vi "acq.Video.vi"(7 "DVR":T3, 8 "error in":errorcluster, 9 "video":T2=TRUE caption="Save Video", 10 "buffer in":u16[][](array[numeric])) -> (0 "error out":errorcluster, 2 "AVI Refnum":T1)   [LabVIEW 2020]
uses:
  _controls/data.ctl
  camera/camera.lvclass
  _controls/data.ref.ctl
  <vilib>/vision/Image Controls.llb/IMAQ Image.ctl
  _controls/state.ctl
  _controls/data.vars.ctl
  _controls/flip.ctl
  _controls/checkbox.ctl
  <vilib>/vision/Avi.llb/IMAQ AVI2 Refnum.ctl
  pix.sgl.CalcPercentiles.sgl.vi
  pix.sgl.CalcPercentiles.vi
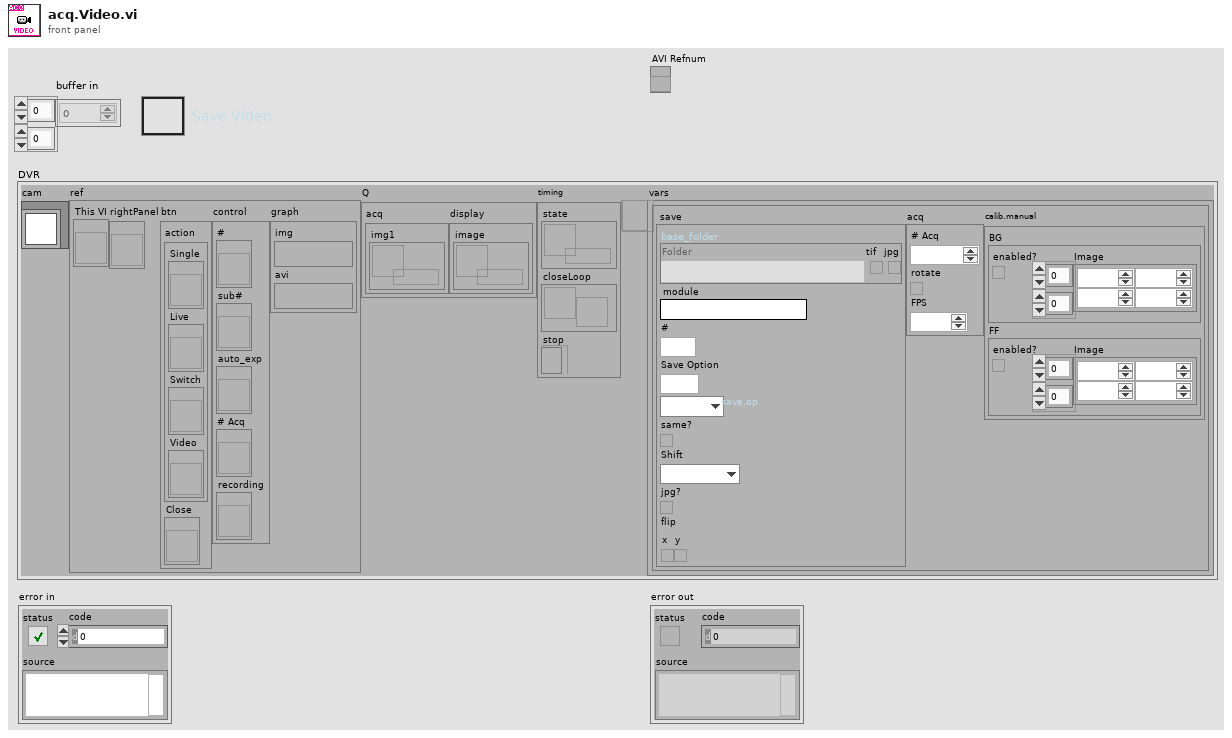
[diagram p1: front panel]
types:
  T1 = typedef "IMAQ AVI2 Refnum.ctl" = refnum<k20>
  T2 = typedef "checkbox.ctl" = bool
  T3 = typedef "data.ctl" = cluster{"cam":refnum<class "camera.lvclass">, "ref":T4, "Q":cluster{"acq":cluster{"img1":refnum<queue>}, "display":cluster{"image":refnum<queue>}}, "timing":cluster{"state":refnum<queue>, "closeLoop":refnum<notifier>, "stop":refnum<k4>}, "vars":refnum<data-value>}
  T4 = typedef "data.ref.ctl" = cluster{"This VI":refnum<vi>, "rightPanel":refnum<vi>, "btn":cluster{"action":cluster{"Single":refnum<vi>, "Live":refnum<vi>, "Switch":refnum<vi>, "Video":refnum<vi>}, "Close":refnum<vi>}, "control":cluster{"#":refnum<vi>, "sub#":refnum<vi>, "auto_exp":refnum<vi>, "# Acq":refnum<vi>, "recording":refnum<vi>}, "graph":cluster{"img":T5, "avi":T5}}
  T5 = typedef "IMAQ Image.ctl" = refnum<image>
  T6 = typedef "data.vars.ctl" = cluster{"save":cluster{"base_folder":cluster{"Folder":path, "tif":bool, "jpg":bool}, "module":string, "#":u32, "sub#":u8, "save.op":enum16{"Full", "Light"}, "same?":bool, "Shift":enum16{"Single", "Leapfrog"}, "jpg?":bool, "flip":T7}, "acq":cluster{"# Acq":u16, "rotate":bool, "FPS":dbl}, "calib.manual":cluster{"BG":cluster{"Image":u16[][], "enabled?":bool}, "FF":cluster{"Image":u16[][], "enabled?":bool}}}
  T7 = typedef "flip.ctl" = cluster{"x":bool, "y":bool}
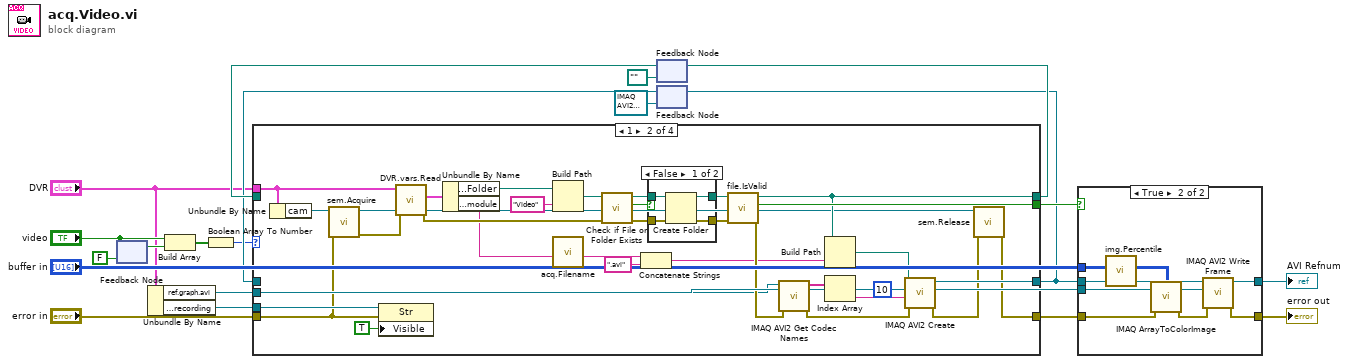
[diagram p0: block diagram]
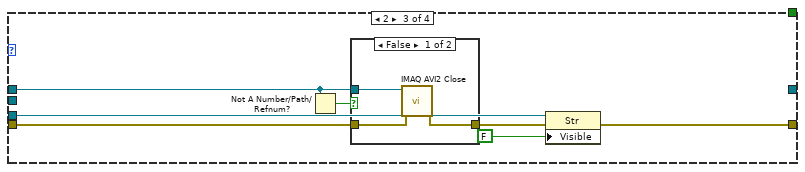
[diagram p4: hidden frame]
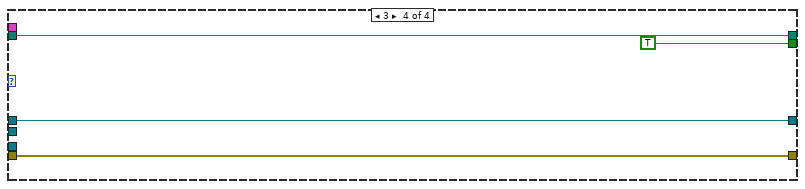
[diagram p6: hidden frame]
diagram:
  n1 = feedback #1(T2 FALSE ("video")) -> (w8:T2)
  n2 = feedback-in #1("video") -> ()
  n3 = Unbundle By Name("DVR") -> ("ref.graph.avi"=w4:T5, "ref.control.recording"=w1:refnum<vi>)
  n4 = Build Array("video", w8) -> (w7:T2[])
  n5 = Boolean Array To Number(Boolean array=w7) -> (number=w6:u32)
  n6 = feedback #2(path "" ("dup path")) -> (w13:path)
  n7 = feedback #3(T1 refnum ("AVI Refnum")) -> (w10:T1)
  n8 = case shown="1" w6 {
    tunnel: "DVR" -> [_ w27 _ _]
    tunnel: [_ w47 _ TRUE ("valid file/folder?")] -> w15
    tunnel: "error in" -> [w22 w28 w68 w73]
    tunnel: w13 -> [w23 _ _ w76]
    tunnel: [w23 w32 _ w76] -> w14
    tunnel: [w21 w41 _ w74] -> w9
    tunnel: [w22 w24 w64 w73] -> w11
    tunnel: w10 -> [w21 _ w66 w74]
    tunnel: w4 -> [_ w35 _ _]
    tunnel: w1 -> [_ w30 w62 _]
    frame Default {
    }
    frame 1 {
      n9 = Unbundle By Name(w27) -> ("cam"=w26:refnum<class "camera.lvclass">)
      n10 = call "sem.Acquire.vi"("error in"=w28, "camera.nit in"=w26) -> ("error out"=w29:errorcluster)  [unwired: 9 in]
      n11 = property class="Str"(reference=w30, error in=w28, "Visible"=TRUE) -> ()  [unwired: 2 out]
      n12 = call "DVR.vars.Read.vi"("error in"=w29, "DVR.state"=w27) -> ("error out"=w48:errorcluster, "vars"=w55:T6)  [unwired: 8 in]
      n13 = Unbundle By Name(w55) -> ("save.base_folder.Folder"=w49:path, "save.module"=w36:string)
      n14 = Build Path(base path=w49, name or relative path="Video" ("foldernme")) -> (appended path=w46:path)
      n15 = call "acq.Filename.vi"("module"=w36) -> ("filename"=w37:string)  [unwired: 10 in]
      n16 = call <vilib>:"Check if File or Folder Exists.vi"("error in (no error)"=w48, "path"=w46) -> ("error out"=w54:errorcluster, "file or folder exists?"=w52:bool, "dup path"=w50:path)  [unwired: 7 in]
      n17 = Concatenate Strings(w37, ".avi" ("string")) -> (w34:string)
      n18 = case shown="False" w52 {
        tunnel: w50 -> [w59 w60]
        tunnel: w54 -> [w58 w61]
        tunnel: [w57 w61] -> w53
        tunnel: [w56 w60] -> w51
        frame False {
          n19 = Create Folder(path (use dialog)=w59, error in=w58) -> (created path=w56:path, error out=w57:errorcluster)  [unwired: 1 in, 1 out]
        }
        frame True {
        }
      }
      n20 = call "file.IsValid.vi"("error in (no error)"=w53, "path"=w51) -> ("error out"=w38:errorcluster, "valid file/folder?"=w47:bool, "dup path"=w32:path)  [unwired: 7 in]
      n21 = call "IMAQ AVI2 Get Codec Names"("error in (no error)"=w38, "Image"=w35) -> ("error out"=w42:errorcluster, "Codec Names"=w43:string[])  [unwired: 8 in]
      n22 = Build Path(base path=w32, name or relative path=w34) -> (appended path=w40:path)
      n23 = Index Array(array=w43) -> (element=w44:string)  [unwired: 1 in]
      n24 = call "IMAQ AVI2 Create"("error in (no error)"=w42, "Codec"=w44, "Frames Per Second"=u32 10, "AVI Path"=w40) -> ("error out"=w25:errorcluster, "AVI Refnum"=w41:T1)  [unwired: 6 in]
      n25 = call "sem.Release.vi"("error in"=w25, "camera.nit in"=w26) -> ("error out"=w24:errorcluster)  [unwired: 9 in]
    }
    frame 2 {
      n26 = Not A Number/Path/Refnum?(number/path/refnum=w66) -> (NaN/Path/Refnum?=w65:bool)
      n27 = case shown="False" w65 {
        tunnel: w68 -> [w71 w72]
        tunnel: [w70 w72] -> w67
        tunnel: w66 -> [w69 _]
        frame False {
          n28 = call "IMAQ AVI2 Close"("error in (no error)"=w71, "AVI Refnum"=w69) -> ("error out"=w70:errorcluster)  [unwired: 9 in]
        }
        frame True {
        }
      }
      n29 = property class="Str"(reference=w62, error in=w67, "Visible"=FALSE) -> (error out=w64:errorcluster)  [unwired: 1 out]
    }
    frame 3 {
    }
  }
  n30 = feedback-in #2(w14) -> ()
  n31 = feedback-in #3(w9) -> ()
  n32 = case shown="True" w15 {
    tunnel: "buffer in" -> [_ w79]
    tunnel: w9 -> [_ w85]
    tunnel: w11 -> [w77 w84]
    tunnel: [w77 w82] -> w17
    tunnel: [_ w81] -> w16
    tunnel: w4 -> [_ w80]
    frame False {
    }
    frame True {
      n33 = call "img.Percentile.vi"("U16 image in"=w79) -> ("U32 image out"=w78:u32[][])  [unwired: 10 in]
      n34 = call "IMAQ ArrayToColorImage"("Image Pixels (U32)"=w78, "Image"=w80, "error in (no error)"=w84) -> ("Image Out"=w86:T5, "error out"=w83:errorcluster)  [unwired: 2 in]
      n35 = call "IMAQ AVI2 Write Frame"("error in (no error)"=w83, "Image"=w86, "AVI Refnum"=w85) -> ("error out"=w82:errorcluster, "AVI Refnum (duplicate)"=w81:T1)  [unwired: 6 in, 1 out]
    }
  }
  "error out" <- w17
  "AVI Refnum" <- w16
